vi "运维调试_CODCr.vi"() -> ()   [LabVIEW 2016, in "CodCr.lvlib"]
uses:
  CodCr.lvlib
  <vilib>/Utility/miscctls.llb/LVPointTypeDef.ctl
  <vilib>/Plasmionique/MB Master/MB_Master_Serial/MB_Master_Serial.lvclass
  C:/Program Files (x86)/National Instruments/LabVIEW 2016/vi.lib/Plasmionique/MB Master/MB_Master/MB_Master.lvclass
  <vilib>/Plasmionique/MB Master/MB Master.lvlib
  <vilib>/ptbypt/NI_PtbyPt.lvlib
panel:
  out "COM口":string
  in  "空白测试":bool
  in  "隐藏按钮":bool
  in  "写入消解温度时长":bool
  in  "保存KB值":bool
  out "source":string
  in  "标样核查":bool
  out "启动时间":timestamp format="%<%Y/%m/%d %H:%M:%S>T"
  out "主循环次数":i32
  out "status":bool
  out "启动测量模式":T1(ring)
  out "曲线斜率B":sgl format="%#_10g"
  out "曲线斜率K":sgl format="%#_10g"
  out "量程上限":sgl
  out "量程下限":sgl
  out "消解时长":u16
  out "消解温度":u16
  out "测量精度":u16
  out "测量结果":sgl
  out "标样参考值":sgl
  out "量程":u16
  out "工作状态":T1(ring)
  out "仪器时间":timestamp format="%<%X\n%x>T"
  out "关键参数区":T2
  out "状态告警区":T3
  out "测量数据区":T4 {"单位" items=["ug/L", "mg/L", "ppm", "mg/m3", "cm", "ppb", "ug/m3", "%", "nmol/mol", "umol/mol", "MPN/L", "MPN/100ml", "ng/m3", "NTU", "无量纲", "ms/cm", "us/cm", "℃", "mV", "万个/L"]}
  out "系统时间":timestamp format="%<%Y/%m/%d %H:%M:%S>T"
  in  "VISA Resource":refnum<visa-resource-name>="COM9"
  out "Registers":u16[](array[numeric])
  in  "枚举":enum16{"读取", "写入", "读取参数"}(ring)
  in  "停止":bool
  in  "校时":bool
  in  "标样校准":bool
  in  "空白校准":bool
  in  "零点核查":bool
  in  "跨度核查":bool
  in  "水样测试":bool
  in  "返回":bool
  in  "设置":bool
  # "mg/L"
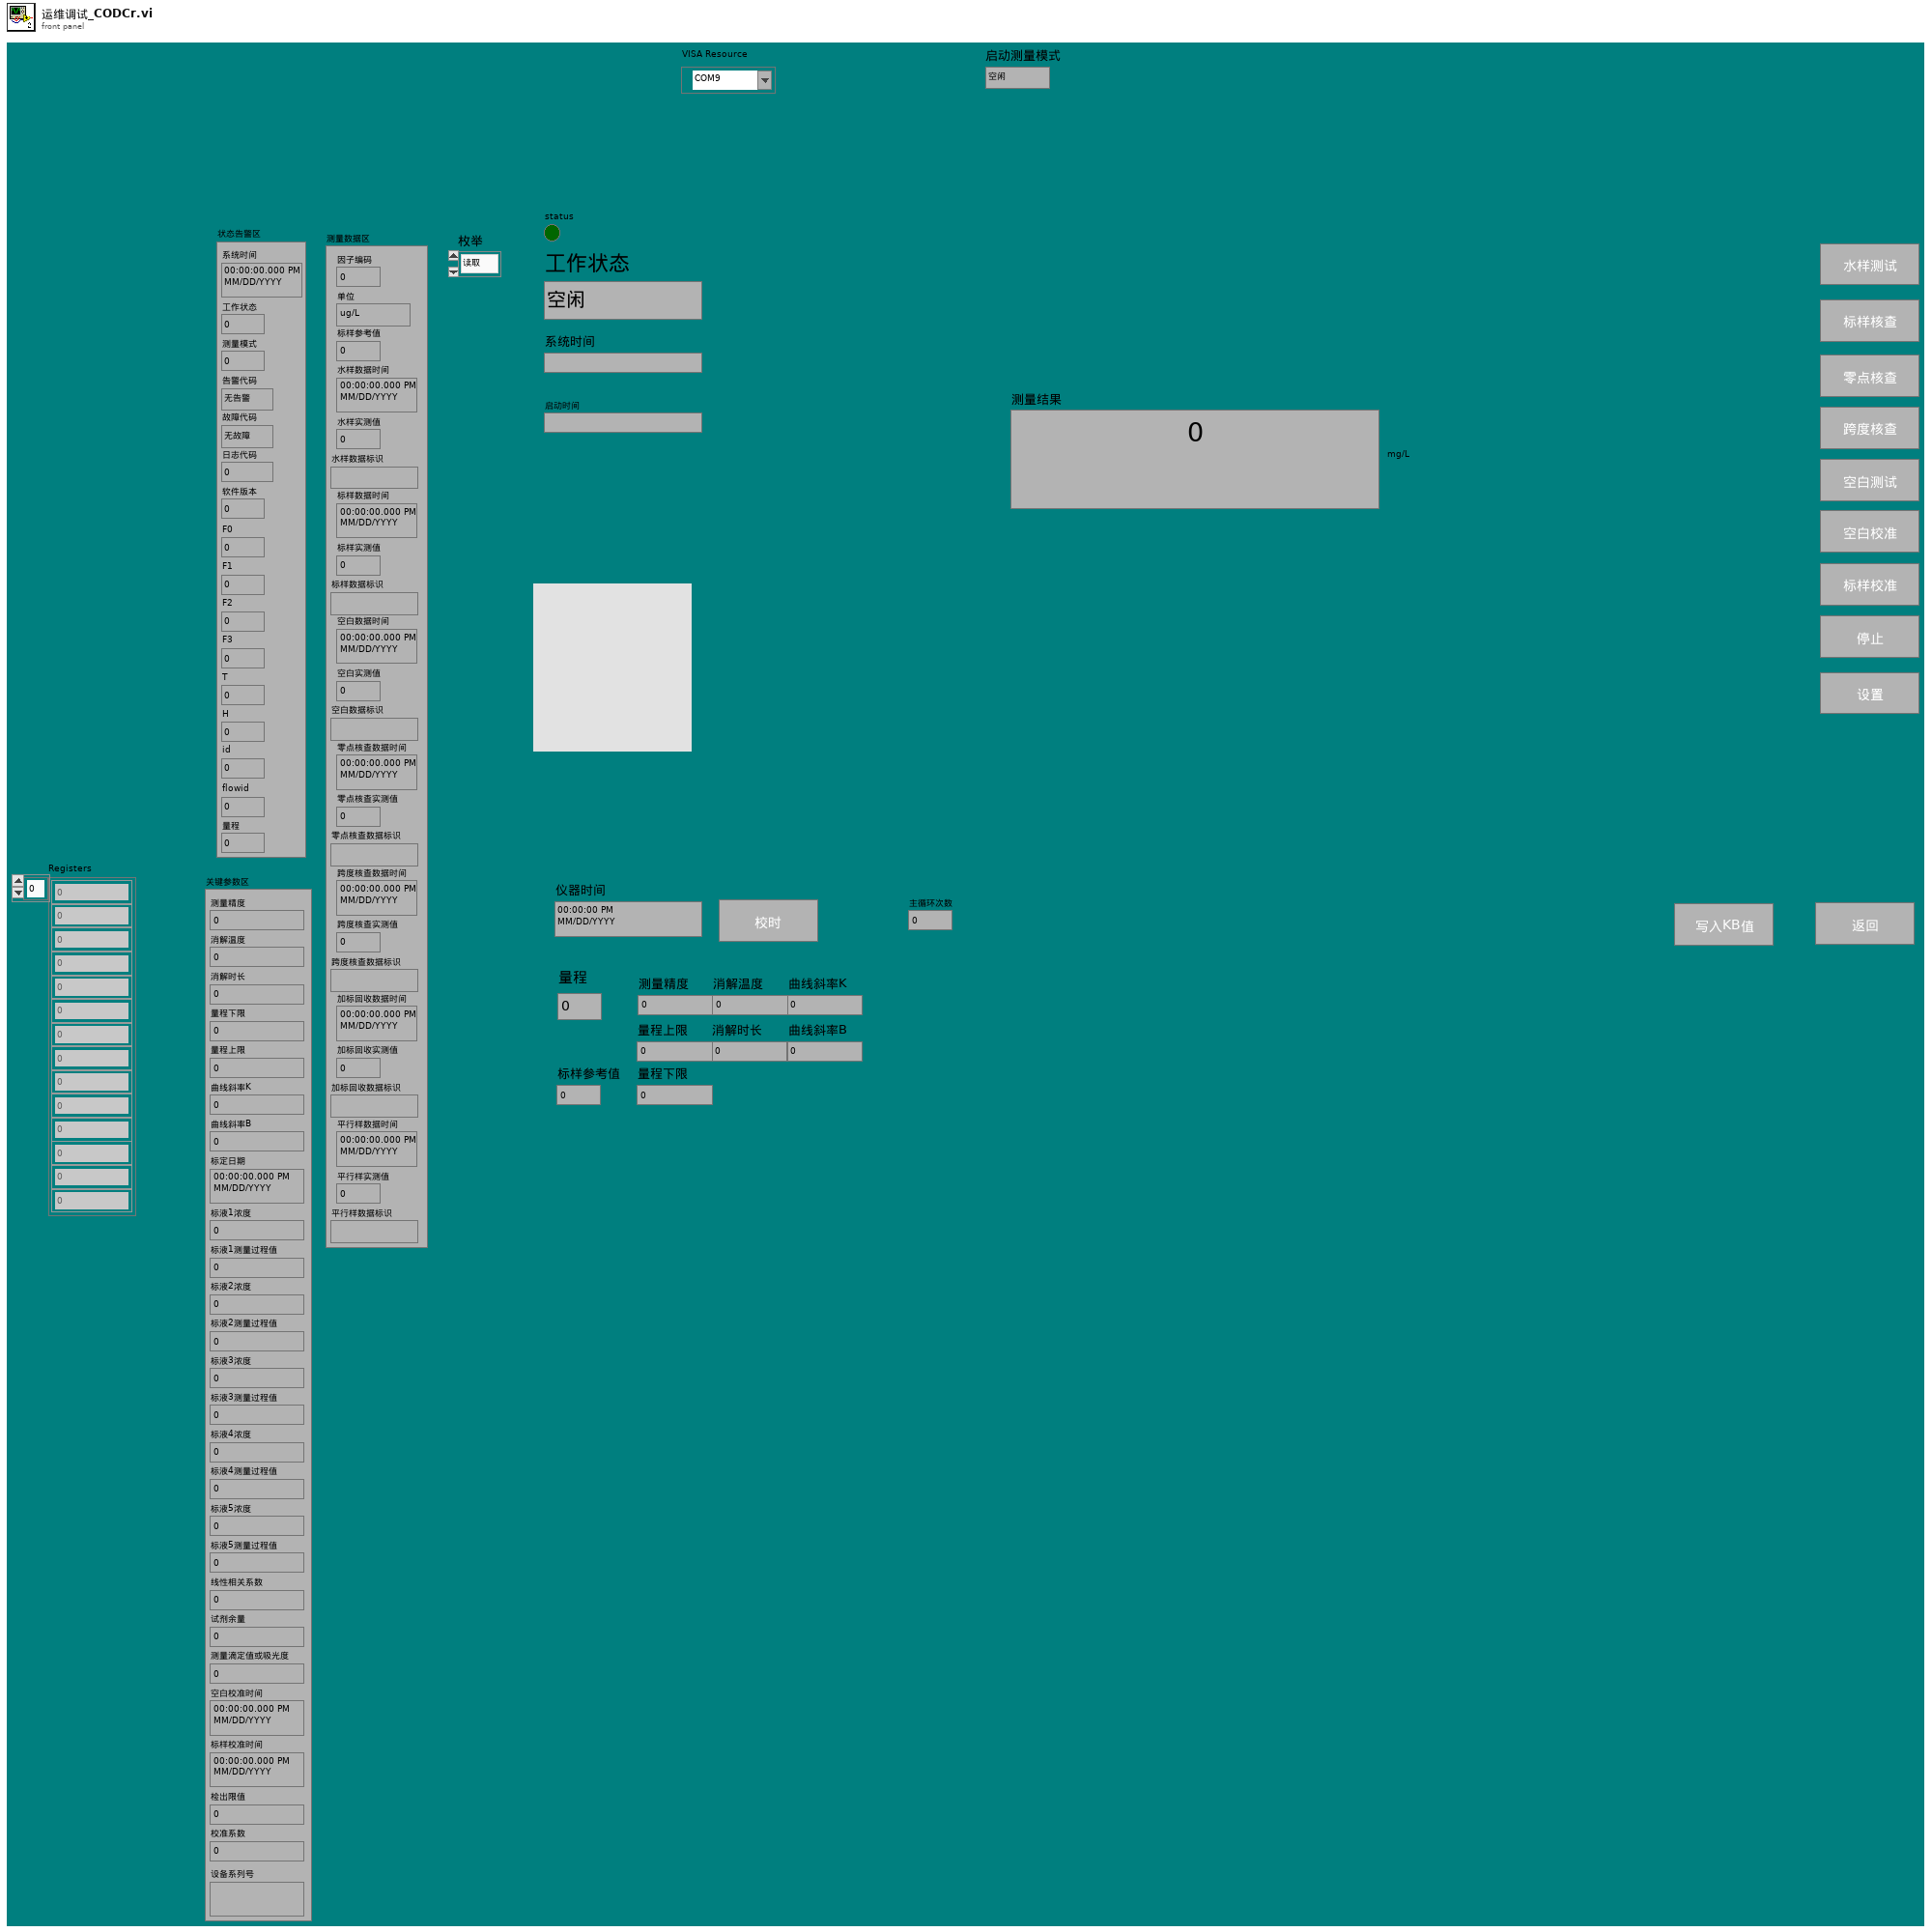
[diagram p1: front panel]
types:
  T1 = enum16{"空闲", "水样测试", "标样核查", "零点核查", "跨度核查", "空白测试", "平行样测试", "加标回收", "空白校准", "标样校准", "初始化（清洗）"}
  T2 = cluster{"测量精度":u16, "消解温度":u16, "消解时长":u16, "量程下限":sgl, "量程上限":sgl, "曲线斜率K":sgl, "曲线斜率B":sgl, "标定日期":timestamp, "标液1浓度":sgl, "标液1测量过程值":sgl, "标液2浓度":sgl, "标液2测量过程值":sgl, "标液3浓度":sgl, "标液3测量过程值":sgl, "标液4浓度":sgl, "标液4测量过程值":sgl, "标液5浓度":sgl, "标液5测量过程值":sgl, "线性相关系数":sgl, "试剂余量":u32, "测量滴定值或吸光度":sgl, "空白校准时间":timestamp, "标样校准时间":timestamp, "检出限值":sgl, "校准系数":sgl, "设备系列号":string}
  T3 = cluster{"系统时间":timestamp, "工作状态":u16, "测量模式":u16, "告警代码":enum16{"无告警", "缺试剂告警", "缺水样告警", "缺蒸馏水告警", "缺标液告警", "仪表漏液告警", "标定异常告警", "超量程告警", "加热异常", "低试剂预警", "超上限告警", "超下限告警", "仪表内部其他异常", "滴定异常告警", "电极异常告警", "量程切换告警", "参数设置告警", "PH电极电位异常", "电导率电极异常", "浊度光度异常", "溶解氧电极异常", "溶解氧光强异常", "温度异常告警", "PH异常告警", "溶解氧异常告警", "电导率异常告警", "浊度异常告警", "叶绿素异常告警", "藻密度异常告警", "蓝绿藻异常告警", "ORP异常告警", "氨氮异常告警", "清洁刷异常告警", "SD卡异常告警", "蓝牙异常告警", "Wifi异常告警", "流程异常告警"}, "故障代码":enum16{"无故障", "电机故障", "温度故障", "通讯故障", "滴定故障"}, "日志代码":u16, "软件版本":u16, "F0":sgl, "F1":sgl, "F2":sgl, "F3":sgl, "T":sgl, "H":sgl, "id":u16, "flowid":u16, "量程":u16}
  T4 = cluster{"因子编码":u32, "单位":u16, "标样参考值":sgl, "水样数据时间":timestamp, "水样实测值":sgl, "水样数据标识":string, "标样数据时间":timestamp, "标样实测值":sgl, "标样数据标识":string, "空白数据时间":timestamp, "空白实测值":sgl, "空白数据标识":string, "零点核查数据时间":timestamp, "零点核查实测值":sgl, "零点核查数据标识":string, "跨度核查数据时间":timestamp, "跨度核查实测值":sgl, "跨度核查数据标识":string, "加标回收数据时间":timestamp, "加标回收实测值":sgl, "加标回收数据标识":string, "平行样数据时间":timestamp, "平行样实测值":sgl, "平行样数据标识":string}
  T5 = cluster{"baud rate (bps)":u32, "stop bits":u16, "parity":u16, "flow control":u16, "timeout":u32, "retries":i32}
  T6 = cluster{"starting address":u16, "number of holding registers":u16}
  T7 = typedef "LVPointTypeDef.ctl" = cluster{"Horizontal":i16, "Vertical":i16}
  T8 = cluster{"时间标识":timestamp, "监测值":sgl, "单位":u16, "数据标识":string, "因子编码":u32, "标样参考值":sgl, "F0":sgl, "F1":sgl, "F2":sgl, "F3":sgl, "温度":sgl, "湿度":sgl, "量程标识":string}
  T9 = cluster{"系统时间":timestamp, "工作状态":enum16{"空闲", "水样测试", "标样核查", "零点核查", "跨度核查", "空白测试", "平行样测试", "加标回收", "空白校准", "标样校准", "初始化（清洗）"}, "测量模式":enum16{"待机", "连续模式", "周期模式", "定点模式", "受控模式", "手动模式"}, "告警代码":enum16{"无告警", "缺试剂告警", "缺水样告警", "缺蒸馏水告警", "缺标液告警", "仪表漏液告警", "标定异常告警", "超量程告警", "加热异常", "低试剂预警", "超上限告警", "超下限告警", "仪表内部其他异常", "滴定异常告警", "电极异常告警", "量程切换告警", "参数设置告警", "PH电极电位异常", "电导率电极异常", "浊度光度异常", "溶解氧电极异常", "溶解氧光强异常", "温度异常告警", "PH异常告警", "溶解氧异常告警", "电导率异常告警", "浊度异常告警", "叶绿素异常告警", "藻密度异常告警", "蓝绿藻异常告警", "ORP异常告警", "氨氮异常告警", "清洁刷异常告警", "SD卡异常告警", "蓝牙异常告警", "Wifi异常告警", "流程异常告警"}, "故障代码":enum16{"无故障", "电机故障", "温度故障", "通讯故障", "滴定故障"}, "日志代码":u16, "软件版本":u16, "F0":sgl, "F1":sgl, "F2":sgl, "F3":sgl, "T":sgl, "H":sgl, "id":u16, "flowid":u16, "量程":u16}
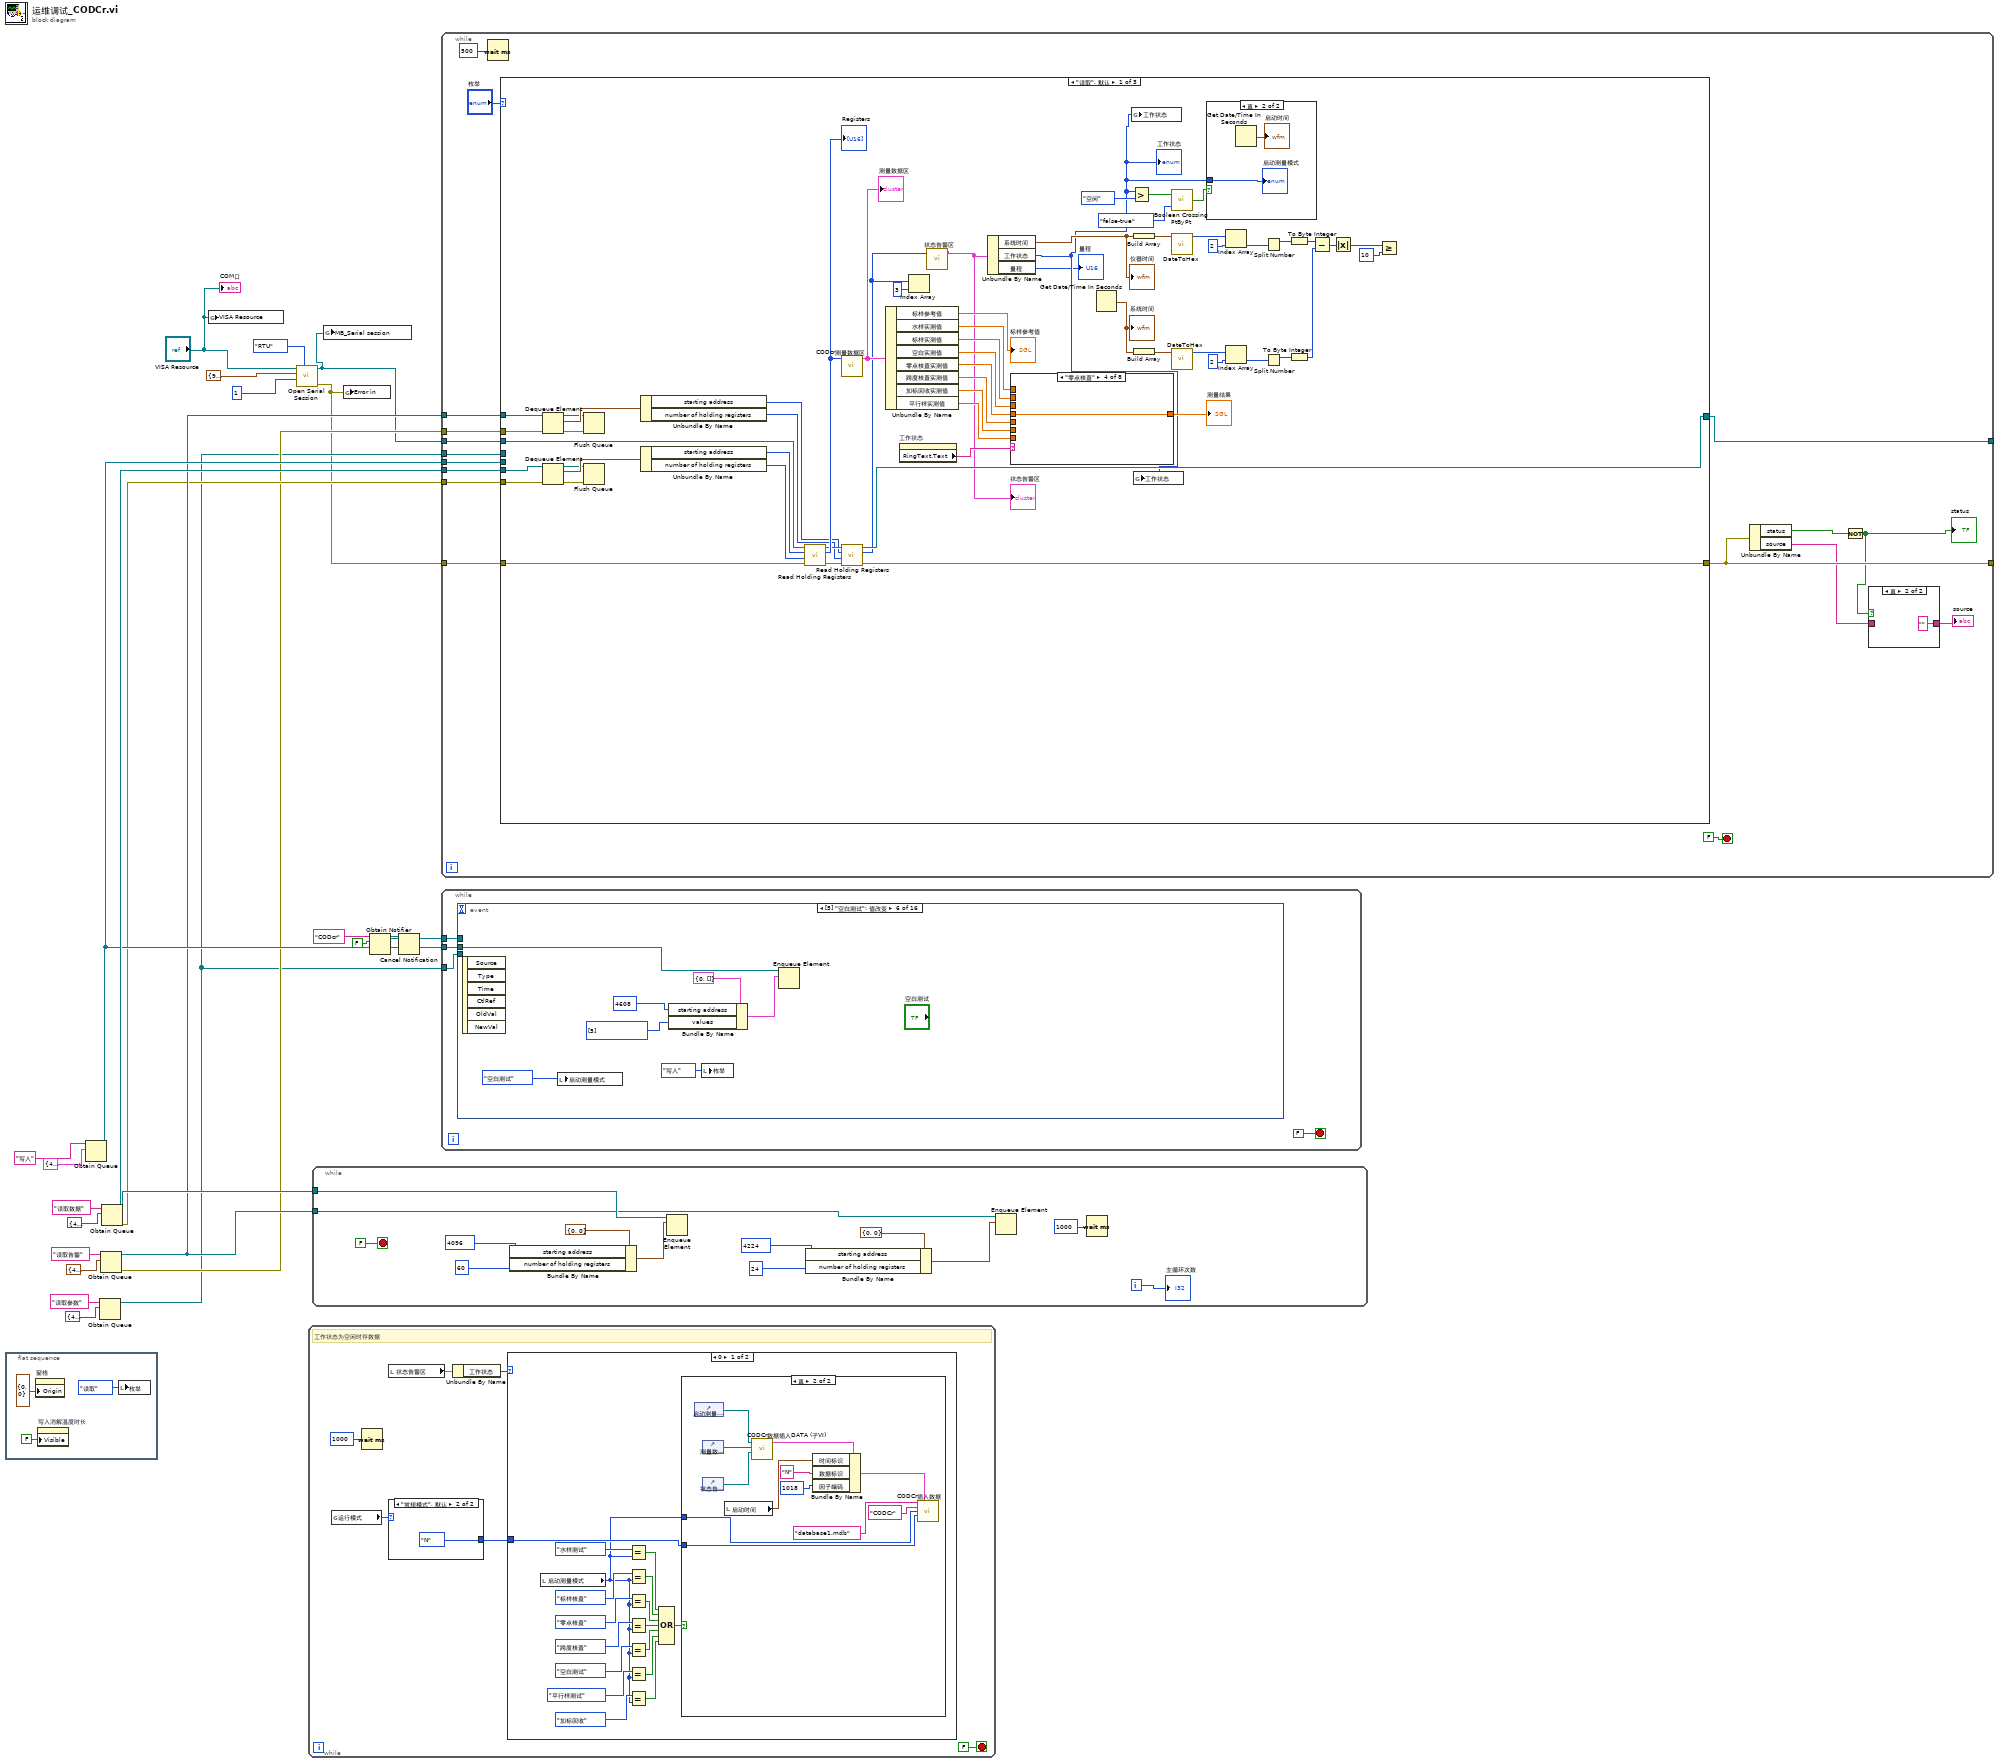
[diagram p0: block diagram]
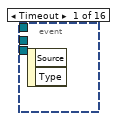
[diagram p2: hidden frame]
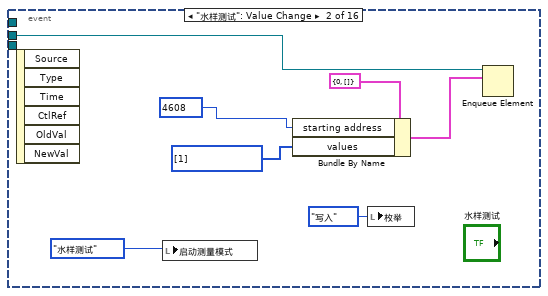
[diagram p3: hidden frame]
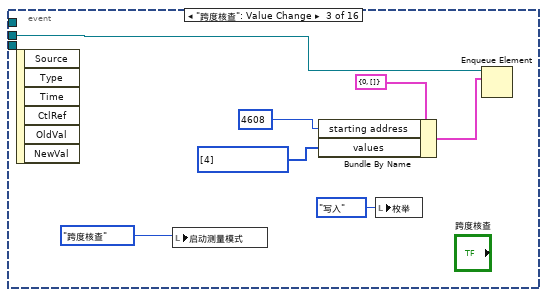
[diagram p4: hidden frame]
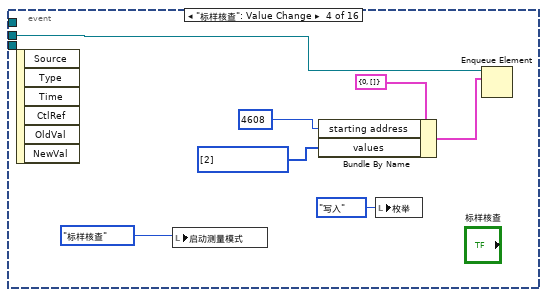
[diagram p5: hidden frame]
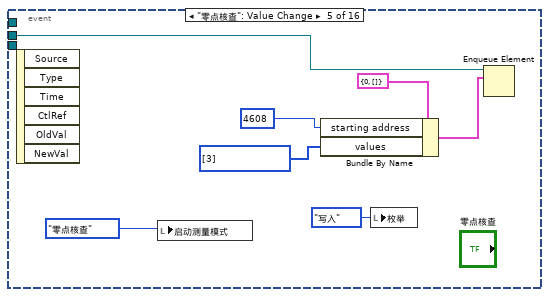
[diagram p6: hidden frame]
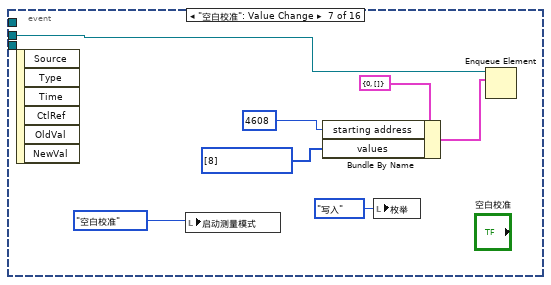
[diagram p7: hidden frame]
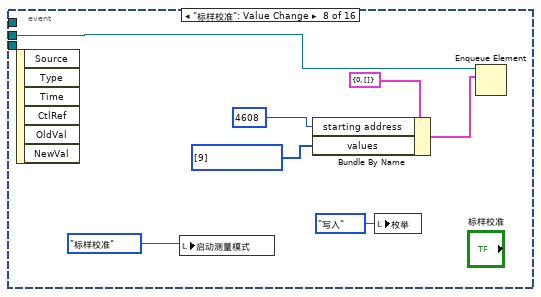
[diagram p8: hidden frame]
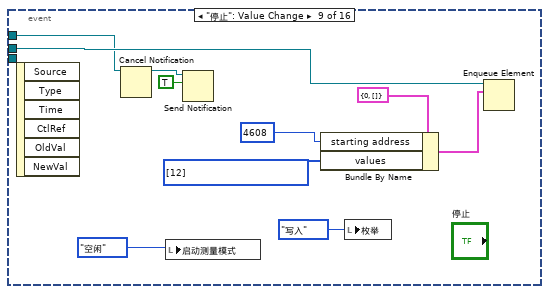
[diagram p9: hidden frame]
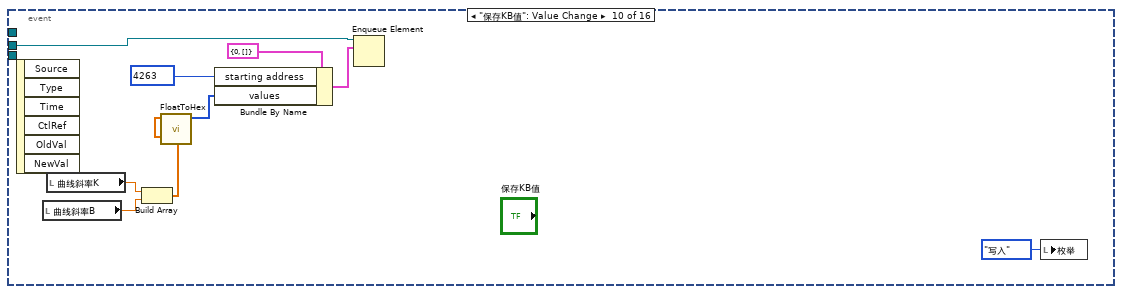
[diagram p10: hidden frame]
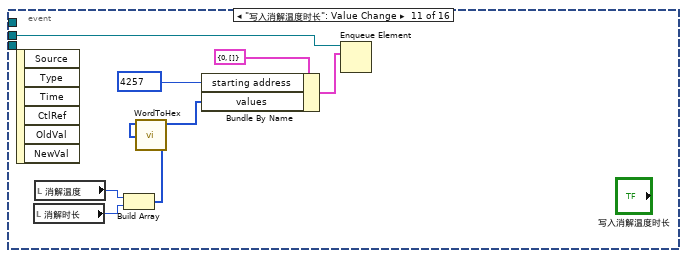
[diagram p11: hidden frame]
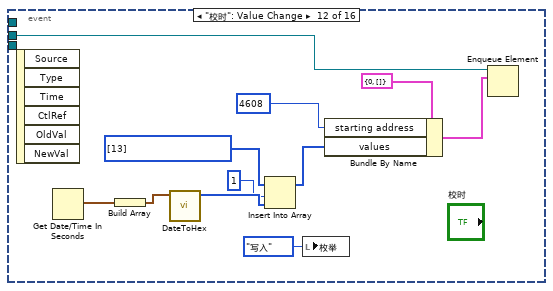
[diagram p12: hidden frame]
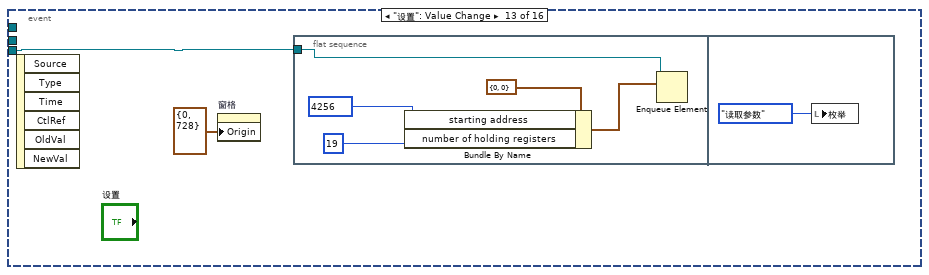
[diagram p13: hidden frame]
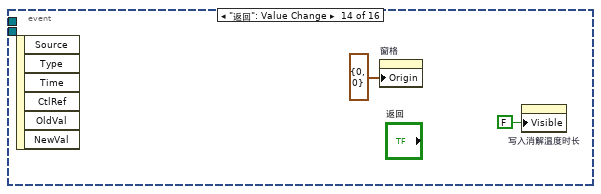
[diagram p14: hidden frame]
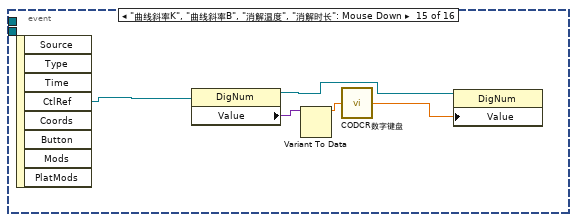
[diagram p15: hidden frame]
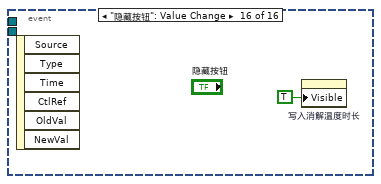
[diagram p16: hidden frame]
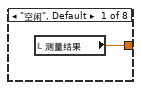
[diagram p18: hidden frame]
diagram:
  n1 = flat-sequence {
    frame #0 {
      n2 = property on="窗格" class="Pane"("Origin"=T7 {"Horizontal"=0, "Vertical"=0} ("原点")) -> ()  [unwired: 2 in, 2 out]
      n3 = property on="写入消解温度时长" class="Bool"("Visible"=FALSE ("可见")) -> ()  [unwired: 2 in, 2 out]
      n4 = local write "枚举"(enum16{"读取", "写入", "读取参数"}."读取" ("枚举")) -> ()
    }
  }
  n5 = Obtain Queue(name (unnamed)="写入" ("名称（未命名）"), element data type=cluster{"starting address":u16, "values":u16[]} {"starting address"=4096, "values"=[]}) -> (queue out=w16:refnum<queue>)  [unwired: 3 in, 2 out]
  n6 = Obtain Queue(name (unnamed)="读取参数" ("名称（未命名）"), element data type=T6 {"starting address"=4096, "number of holding registers"=100}) -> (queue out=w4:refnum<queue>)  [unwired: 3 in, 2 out]
  n7 = Obtain Queue(name (unnamed)="读取告警" ("名称（未命名）"), element data type=T6 {"starting address"=4096, "number of holding registers"=100}) -> (queue out=w13:refnum<queue>, error out=w9:errorcluster)  [unwired: 3 in, 1 out]
  n8 = Obtain Queue(name (unnamed)="读取数据" ("名称（未命名）"), element data type=T6 {"starting address"=4096, "number of holding registers"=100}) -> (queue out=w17:refnum<queue>, error out=w10:errorcluster)  [unwired: 3 in, 1 out]
  n9 = global write "CODcr全局变量.vi" "VISA Resource"("VISA Resource") -> ()
  n10 = call <vilib>:"Open Serial Session.vi"("Mode (RTU)"=enum16{"RTU", "ASCII"}."RTU", "Slave ID"=u8 1, "Serial Config"=T5 {"baud rate (bps)"=9600, "stop bits"=10, "parity"=0, "flow control"=0, "timeout"=1000, "retries"=1}, "VISA Resource"="VISA Resource") -> ("Error out"=w1:errorcluster, "MB_Serial session"=w2:refnum<class "MB_Master_Serial.lvclass">)  [unwired: 6 in]
  n11 = while "While循环" {
    stop <- FALSE stop-if-true
    # "工作状态为空闲时存数据"
    n12 = global read "系统变量.vi" "运行模式"() -> (w29:enum16{"维护模式", "常规模式", "应急模式", "质控模式"})
    n13 = Wait (ms)(milliseconds to wait=u32 1000 ("等待时间（毫秒）")) -> ()  [unwired: 1 out]
    n14 = local read "状态告警区"() -> (w31:T3)
    n15 = case shown="\"常规模式\", 默认" w29 {
      tunnel: [enum16{"N", "M"}."M" ("数据类型") enum16{"N", "M"}."N" ("数据类型")] -> w28
      frame "维护模式" {
      }
      frame "常规模式", Default {
      }
    }
    n16 = Unbundle By Name(w31) -> ("工作状态"=w30:u16)
    n17 = case shown="0" w30 {
      tunnel: w28 -> [w52 _]
      frame 0 {
        n18 = local read "启动测量模式"() -> (w44:T1)
        n19 = Equal?(x=T1."水样测试" ("启动测量模式"), y=w44) -> (x = y?=w43:bool)
        n20 = Equal?(x=T1."标样核查" ("启动测量模式"), y=w44) -> (x = y?=w42:bool)
        n21 = Equal?(x=T1."零点核查" ("启动测量模式"), y=w44) -> (x = y?=w41:bool)
        n22 = Equal?(x=T1."跨度核查" ("启动测量模式"), y=w44) -> (x = y?=w40:bool)
        n23 = Equal?(x=T1."空白测试" ("启动测量模式"), y=w44) -> (x = y?=w39:bool)
        n24 = Equal?(x=T1."平行样测试" ("启动测量模式"), y=w44) -> (x = y?=w38:bool)
        n25 = Equal?(x=T1."加标回收" ("启动测量模式"), y=w44) -> (x = y?=w37:bool)
        n26 = Compound Arithmetic op=OR(w43, w42, w41, w40, w39, w38, w37) -> (w36:bool)
        n27 = case shown="真" w36 {
          tunnel: w44 -> [_ w62]
          tunnel: w52 -> [_ w61]
          frame False {
          }
          frame True {
            n28 = control-ref of="启动测量模式"() -> (w60:refnum<vi>)
            n29 = control-ref of="测量数据区"() -> (w59:refnum<vi>)
            n30 = control-ref of="状态告警区"() -> (w58:refnum<vi>)
            n31 = local read "启动时间"() -> (w56:timestamp)
            n32 = call "CODCr数据插入DATA (子VI).vi"("reference 2"=w58, "reference"=w59, "Enum输入"=w60) -> ("data"=w57:T8)  [unwired: 8 in]
            n33 = Bundle By Name(cluster=w57, "时间标识"=w56, "数据标识"="N", "因子编码"=u32 1018) -> (w55:T8)
            n34 = call "CODCr插入数据.vi"("database"="database1.mdb", "data"=w55, "table"="CODCr", "测量模式"=w62, "数据类型"=w61) -> ()  [unwired: 10 in, 1 out]
          }
        }
      }
      frame 1, Default {
      }
    }
  }
  n35 = while {
    tunnel: w17 -> [w75]
    tunnel: w13 -> [w66]
    i -> [w65]
    stop <- FALSE stop-if-true
    n36 = Bundle By Name(cluster=T6 {"starting address"=0, "number of holding registers"=0} ("元素"), "starting address"=u16 4096, "number of holding registers"=u16 60) -> (w73:T6)
    n37 = Enqueue Element(queue=w75, element=w73) -> ()  [unwired: 2 in, 3 out]
    n38 = Bundle By Name(cluster=T6 {"starting address"=0, "number of holding registers"=0} ("元素"), "starting address"=u16 4224, "number of holding registers"=u16 24) -> (w67:T6)
    n39 = Enqueue Element(queue=w66, element=w67) -> ()  [unwired: 2 in, 3 out]
    n40 = Wait (ms)(milliseconds to wait=u32 1000 ("等待时间（毫秒）")) -> ()  [unwired: 1 out]
    "主循环次数" <- w65
  }
  n41 = global write "CODcr全局变量.vi" "MB_Serial session"(w2) -> ()
  n42 = global write "CODcr全局变量.vi" "Error in"(w1) -> ()
  n43 = Obtain Notifier(name (unnamed)="CODcr" ("名称（未命名）"), notification data type=FALSE) -> (notifier out=w5:refnum<notifier>)  [unwired: 2 in, 2 out]
  n44 = Cancel Notification(0:w5) -> (8:w6:refnum<notifier>)  [unwired: 1 in, 2 out]
  n45 = while {
    tunnel: w16 -> [w91]
    tunnel: w17 -> [w90]
    tunnel: w13 -> [w89]
    tunnel: w4 -> [w88]
    tunnel: w10 -> [w86]
    tunnel: w9 -> [w85]
    tunnel: w1 -> [w84]
    tunnel: [w82] -> _
    tunnel: w2 -> [w92]
    tunnel: [w87] -> _
    stop <- FALSE stop-if-true
    n46 = Wait (ms)(milliseconds to wait=u32 500 ("等待时间（毫秒）")) -> ()  [unwired: 1 out]
    n47 = case shown="\"读取\", 默认" "枚举" {
      tunnel: w92 -> [w154 w171 w194]
      tunnel: w84 -> [w130 w170 w193]
      tunnel: w91 -> [_ w169 _]
      tunnel: w90 -> [w153 _ _]
      tunnel: w89 -> [w148 _ _]
      tunnel: w88 -> [_ _ w195]
      tunnel: [w129 w165 w183] -> w82
      tunnel: [w111 w166 w184] -> w87
      tunnel: w86 -> [w105 _ _]
      tunnel: w85 -> [w102 _ _]
      frame "读取", Default {
        n48 = Dequeue Element(queue=w148, error in (no error)=w102) -> (queue out=w104:refnum<queue>, element=w147:T6, error out=w103:errorcluster)  [unwired: 1 in, 1 out]
        n49 = Dequeue Element(queue=w153, error in (no error)=w105) -> (queue out=w107:refnum<queue>, element=w152:T6, error out=w106:errorcluster)  [unwired: 1 in, 1 out]
        n50 = Flush Queue(queue=w104, error in (no error)=w103) -> ()  [unwired: 3 out]
        n51 = Flush Queue(queue=w107, error in (no error)=w106) -> ()  [unwired: 3 out]
        n52 = Unbundle By Name(w147) -> ("starting address"=w144:u16, "number of holding registers"=w143:u16)
        n53 = Unbundle By Name(w152) -> ("starting address"=w151:u16, "number of holding registers"=w150:u16)
        n54 = call <vilib>:"Read Holding Registers.vi"("error in (no error)"=w130, "quantity"=w150, "starting address"=w151, "MB session in"=w154) -> ("error out"=w145:errorcluster, "Registers"=w149:u16[], "MB session out"=w146:refnum<class "MB_Master_Serial.lvclass">)  [unwired: 5 in]
        "Registers" <- w149
        n55 = call "CODcr测量数据区.vi"("数组"=w149) -> ("测量数据区"=w142:T4)  [unwired: 10 in]
        "测量数据区" <- w142
        n56 = call <vilib>:"Read Holding Registers.vi"("error in (no error)"=w145, "quantity"=w143, "starting address"=w144, "MB session in"=w146) -> ("error out"=w129:errorcluster, "Registers"=w98:u16[], "MB session out"=w111:refnum<class "MB_Master_Serial.lvclass">)  [unwired: 5 in]
        n57 = Unbundle By Name(w142) -> ("标样参考值"=→"标样参考值":sgl, "水样实测值"=w138:sgl, "标样实测值"=w136:sgl, "空白实测值"=w133:sgl, "零点核查实测值"=w135:sgl, "跨度核查实测值"=w134:sgl, "加标回收实测值"=w131:sgl, "平行样实测值"=w132:sgl)
        n58 = property on="工作状态" class="Enum (严格)"() -> ("RingText.Text"=w139:string)  [unwired: 2 in, 2 out]
        n59 = Index Array(array=w98, index=3 ("索引")) -> ()  [unwired: 1 out]
        n60 = call "状态告警区.vi"("数组"=w98) -> ("状态告警区"=w97:T9)  [unwired: 10 in]
        "状态告警区" <- w97
        n61 = Unbundle By Name(w97) -> ("系统时间"=w112:timestamp, "工作状态"=w100:T1, "量程"=→"量程":u16)
        "仪器时间" <- w112
        "工作状态" <- w100
        n62 = case shown="\"零点核查\"" w139 {
          tunnel: w138 -> [_ w156 _ _ _ _ _ _]
          tunnel: [w155 w156 w157 w158 w159 w160 w161 w162] -> w137
          tunnel: w136 -> [_ _ w157 _ _ _ _ _]
          tunnel: w135 -> [_ _ _ w158 _ _ _ _]
          tunnel: w134 -> [_ _ _ _ w159 _ _ _]
          tunnel: w133 -> [_ _ _ _ _ w160 _ _]
          tunnel: w132 -> [_ _ _ _ _ _ w161 _]
          tunnel: w131 -> [_ _ _ _ _ _ _ w162]
          frame "空闲", Default {
            n63 = local read "测量结果"() -> (w155:sgl)
          }
          frame "水样测试" {
          }
          frame "标样核查" {
          }
          frame "零点核查" {
          }
          frame "跨度核查" {
          }
          frame "空白测试" {
          }
          frame "平行样测试" {
          }
          frame "加标回收" {
          }
        }
        "测量结果" <- w137
        n64 = Get Date/Time In Seconds() -> (seconds since 1Jan1904=w114:timestamp)
        "系统时间" <- w114
        n65 = Greater?(x=w100, y=T1."空闲") -> (0:w110:bool)
        n66 = global write "CODcr全局变量.vi" "工作状态"(w100) -> ()
        n67 = Build Array(w112) -> (w128:timestamp[])
        n68 = Build Array(w114) -> (w113:timestamp[])
        n69 = global write "CODCr工作状态.vi" "工作状态"(w100) -> ()
        n70 = call <vilib>:"Boolean Crossing PtByPt.vi"("direction"=enum16{"either", "false-true", "true-false"}."false-true", "input"=w110) -> ("crossing"=w109:bool)  [unwired: 1 in]
        n71 = call "DateToHex.vi"("DATE"=w128) -> ("数组"=w120:u16[])  [unwired: 10 in]
        n72 = call "DateToHex.vi"("DATE"=w113) -> ("数组"=w115:u16[])  [unwired: 10 in]
        n73 = case shown="真" w109 {
          tunnel: w100 -> [_ w163]
          frame False {
          }
          frame True {
            n74 = Get Date/Time In Seconds() -> (seconds since 1Jan1904=→"启动时间":timestamp)
            "启动测量模式" <- w163
          }
        }
        n75 = Index Array(array=w120, index=2 ("索引")) -> (element=w118:u16)
        n76 = Index Array(array=w115, index=2 ("索引")) -> (element=w117:u16)
        n77 = Split Number(x=w118) -> (hi(x)=w124:u8)  [unwired: 1 out]
        n78 = Split Number(x=w117) -> (hi(x)=w121:u8)  [unwired: 1 out]
        n79 = To Byte Integer(number=w124) -> (8bit integer=w125:i8)
        n80 = To Byte Integer(number=w121) -> (8bit integer=w122:i8)
        n81 = Subtract(x=w125, y=w122) -> (x-y=w123:i8)
        n82 = Absolute Value(x=w123) -> (abs(x)=w126:i8)
        n83 = Greater Or Equal?(x=w126, y=i8 10) -> ()  [unwired: 1 out]
      }
      frame "写入" {
        n84 = flat-sequence {
          tunnel: w171 -> [w179]
          tunnel: w170 -> [w178]
          tunnel: w169 -> [w175]
          tunnel: [w177] -> w168
          tunnel: [w176] -> w167
          tunnel: w168 -> [w181]
          tunnel: w167 -> [w180]
          tunnel: [w181] -> w166
          tunnel: [w180] -> w165
          frame #0 {
            n85 = Dequeue Element(queue=w175) -> (element=w174:cluster{"starting address":u16, "values":u16[]})  [unwired: 2 in, 3 out]
            n86 = Unbundle By Name(w174) -> ("starting address"=w173:u16, "values"=w172:u16[])
            n87 = call <vilib>:"Write Multiple Registers.vi"("error in (no error)"=w178, "values"=w172, "starting address"=w173, "MB session in"=w179) -> ("error out"=w176:errorcluster, "MB session out"=w177:refnum<class "MB_Master_Serial.lvclass">)  [unwired: 6 in]
          }
          frame #1 {
            n88 = local write "枚举"(enum16{"读取", "写入", "读取参数"}."读取" ("枚举")) -> ()
          }
        }
      }
      frame "读取参数" {
        n89 = local write "枚举"(enum16{"读取", "写入", "读取参数"}."读取" ("枚举")) -> ()
        n90 = Dequeue Element(queue=w195, timeout in ms (-1)=1000 ("超时毫秒(-1)")) -> (element=w202:T6)  [unwired: 1 in, 3 out]
        n91 = Unbundle By Name(w202) -> ("starting address"=w201:u16, "number of holding registers"=w200:u16)
        n92 = call <vilib>:"Read Holding Registers.vi"("error in (no error)"=w193, "quantity"=w200, "starting address"=w201, "MB session in"=w194) -> ("error out"=w197:errorcluster, "Registers"=w199:u16[], "MB session out"=w184:refnum<class "MB_Master_Serial.lvclass">)  [unwired: 5 in]
        n93 = call "关键参数区.vi"("数组"=w199) -> ("关键参数区"=w196:T2)  [unwired: 10 in]
        "关键参数区" <- w196
        n94 = Unbundle By Name(w196) -> ("测量精度"=→"测量精度":u16, "消解温度"=→"消解温度":u16, "消解时长"=→"消解时长":u16, "量程下限"=→"量程下限":sgl, "量程上限"=→"量程上限":sgl, "曲线斜率K"=→"曲线斜率K":sgl, "曲线斜率B"=→"曲线斜率B":sgl)
        n95 = call <vilib>:"Clear Errors.vi"("error in (no error)"=w197) -> ("error out"=w183:errorcluster)  [unwired: 5 in, 1 out]
      }
    }
    n96 = Unbundle By Name(w82) -> ("status"=w83:bool, "source"=w80:string)
    n97 = Not(x=w83) -> (.not. x?=w79:bool)
    "status" <- w79
    n98 = case shown="真" w79 {
      tunnel: w80 -> [w95 _]
      tunnel: [w95 "" ("source")] -> w78
      frame False {
      }
      frame True {
      }
    }
    "source" <- w78
  }
  n99 = while {
    tunnel: w16 -> [w205]
    tunnel: w6 -> [w204]
    tunnel: w4 -> [w203]
    stop <- FALSE stop-if-true
    n100 = event shown="[5] \"空白测试\": 值改变" {
      selector: _ -> [_ _ _ _ _ _ _ _ _ _ _ _ _ _ _ _]
      dyn-events: _ -> [_ _ _ _ _ _ _ _ _ _ _ _ _ _ _ _]
      timeout: _ -> [_ _ _ _ _ _ _ _ _ _ _ _ _ _ _ _]
      tunnel: w205 -> [_ w213 w216 w223 w230 w237 w244 w251 w261 w273 w279 w290 _ _ _ _]
      tunnel: w204 -> [_ _ _ _ _ _ _ _ w259 _ _ _ _ _ _ _]
      tunnel: w203 -> [_ _ _ _ _ _ _ _ _ _ _ _ w294 _ _ _]
      event Timeout {
        n101 = event-data() -> ()  [unwired: 1 in, 2 out]
      }
      event "水样测试": Value Change {
        n102 = event-data() -> ()  [unwired: 1 in, 6 out]
        n103 = local write "启动测量模式"(T1."水样测试" ("启动测量模式")) -> ()
        n104 = Bundle By Name(cluster=cluster{"starting address":u16, "values":u16[]} {"starting address"=0, "values"=[]} ("元素"), "starting address"=u16 4608, "values"=u16[] [1]) -> (w211:cluster{"starting address":u16, "values":u16[]})
        n105 = local write "枚举"(enum16{"读取", "写入", "读取参数"}."写入" ("枚举")) -> ()
        n106 = Enqueue Element(queue=w213, element=w211) -> ()  [unwired: 2 in, 3 out]
      }
      event "跨度核查": Value Change {
        n107 = event-data() -> ()  [unwired: 1 in, 6 out]
        n108 = local write "启动测量模式"(T1."跨度核查" ("启动测量模式")) -> ()
        n109 = Bundle By Name(cluster=cluster{"starting address":u16, "values":u16[]} {"starting address"=0, "values"=[]} ("元素"), "starting address"=u16 4608, "values"=u16[] [4]) -> (w219:cluster{"starting address":u16, "values":u16[]})
        n110 = local write "枚举"(enum16{"读取", "写入", "读取参数"}."写入" ("枚举")) -> ()
        n111 = Enqueue Element(queue=w216, element=w219) -> ()  [unwired: 2 in, 3 out]
      }
      event "标样核查": Value Change {
        n112 = event-data() -> ()  [unwired: 1 in, 6 out]
        n113 = local write "启动测量模式"(T1."标样核查" ("启动测量模式")) -> ()
        n114 = Bundle By Name(cluster=cluster{"starting address":u16, "values":u16[]} {"starting address"=0, "values"=[]} ("元素"), "starting address"=u16 4608, "values"=u16[] [2]) -> (w226:cluster{"starting address":u16, "values":u16[]})
        n115 = local write "枚举"(enum16{"读取", "写入", "读取参数"}."写入" ("枚举")) -> ()
        n116 = Enqueue Element(queue=w223, element=w226) -> ()  [unwired: 2 in, 3 out]
      }
      event "零点核查": Value Change {
        n117 = event-data() -> ()  [unwired: 1 in, 6 out]
        n118 = local write "启动测量模式"(T1."零点核查" ("启动测量模式")) -> ()
        n119 = Bundle By Name(cluster=cluster{"starting address":u16, "values":u16[]} {"starting address"=0, "values"=[]} ("元素"), "starting address"=u16 4608, "values"=u16[] [3]) -> (w233:cluster{"starting address":u16, "values":u16[]})
        n120 = local write "枚举"(enum16{"读取", "写入", "读取参数"}."写入" ("枚举")) -> ()
        n121 = Enqueue Element(queue=w230, element=w233) -> ()  [unwired: 2 in, 3 out]
      }
      event "空白测试": Value Change {
        n122 = event-data() -> ()  [unwired: 1 in, 6 out]
        n123 = local write "启动测量模式"(T1."空白测试" ("启动测量模式")) -> ()
        n124 = Bundle By Name(cluster=cluster{"starting address":u16, "values":u16[]} {"starting address"=0, "values"=[]} ("元素"), "starting address"=u16 4608, "values"=u16[] [5]) -> (w240:cluster{"starting address":u16, "values":u16[]})
        n125 = local write "枚举"(enum16{"读取", "写入", "读取参数"}."写入" ("枚举")) -> ()
        n126 = Enqueue Element(queue=w237, element=w240) -> ()  [unwired: 2 in, 3 out]
      }
      event "空白校准": Value Change {
        n127 = event-data() -> ()  [unwired: 1 in, 6 out]
        n128 = local write "启动测量模式"(T1."空白校准" ("启动测量模式")) -> ()
        n129 = Bundle By Name(cluster=cluster{"starting address":u16, "values":u16[]} {"starting address"=0, "values"=[]} ("元素"), "starting address"=u16 4608, "values"=u16[] [8]) -> (w247:cluster{"starting address":u16, "values":u16[]})
        n130 = local write "枚举"(enum16{"读取", "写入", "读取参数"}."写入" ("枚举")) -> ()
        n131 = Enqueue Element(queue=w244, element=w247) -> ()  [unwired: 2 in, 3 out]
      }
      event "标样校准": Value Change {
        n132 = event-data() -> ()  [unwired: 1 in, 6 out]
        n133 = local write "启动测量模式"(T1."标样校准" ("启动测量模式")) -> ()
        n134 = Bundle By Name(cluster=cluster{"starting address":u16, "values":u16[]} {"starting address"=0, "values"=[]} ("元素"), "starting address"=u16 4608, "values"=u16[] [9]) -> (w254:cluster{"starting address":u16, "values":u16[]})
        n135 = local write "枚举"(enum16{"读取", "写入", "读取参数"}."写入" ("枚举")) -> ()
        n136 = Enqueue Element(queue=w251, element=w254) -> ()  [unwired: 2 in, 3 out]
      }
      event "停止": Value Change {
        n137 = event-data() -> ()  [unwired: 1 in, 6 out]
        n138 = Cancel Notification(0:w259) -> (8:w258:refnum<notifier>)  [unwired: 1 in, 2 out]
        n139 = local write "启动测量模式"(T1."空闲" ("启动测量模式")) -> ()
        n140 = Send Notification(notification=TRUE ("通知"), notifier=w258) -> ()  [unwired: 1 in, 2 out]
        n141 = Bundle By Name(cluster=cluster{"starting address":u16, "values":u16[]} {"starting address"=0, "values"=[]} ("元素"), "starting address"=u16 4608, "values"=u16[] [12]) -> (w264:cluster{"starting address":u16, "values":u16[]})
        n142 = local write "枚举"(enum16{"读取", "写入", "读取参数"}."写入" ("枚举")) -> ()
        n143 = Enqueue Element(queue=w261, element=w264) -> ()  [unwired: 2 in, 3 out]
      }
      event "保存KB值": Value Change {
        n144 = event-data() -> ()  [unwired: 1 in, 6 out]
        n145 = local read "曲线斜率B"() -> (w267:sgl)
        n146 = local read "曲线斜率K"() -> (w268:sgl)
        n147 = Build Array(w268, w267) -> (w266:sgl[])
        n148 = call "FloatToHex.vi"("浮点数"=w266) -> ("DCBA整形输出"=w269:u16[])  [unwired: 10 in]
        n149 = Bundle By Name(cluster=cluster{"starting address":u16, "values":u16[]} {"starting address"=0, "values"=[]} ("元素"), "starting address"=u16 4263, "values"=w269) -> (w271:cluster{"starting address":u16, "values":u16[]})
        n150 = Enqueue Element(queue=w273, element=w271) -> ()  [unwired: 2 in, 3 out]
        n151 = local write "枚举"(enum16{"读取", "写入", "读取参数"}."写入" ("枚举")) -> ()
      }
      event "写入消解温度时长": Value Change {
        n152 = event-data() -> ()  [unwired: 1 in, 6 out]
        n153 = local read "消解时长"() -> (w276:u16)
        n154 = local read "消解温度"() -> (w277:u16)
        n155 = Build Array(w277, w276) -> (w275:u16[])
        n156 = call "WordToHex.vi"("WORD"=w275) -> ("数组"=w278:u16[])  [unwired: 10 in]
        n157 = Bundle By Name(cluster=cluster{"starting address":u16, "values":u16[]} {"starting address"=0, "values"=[]} ("元素"), "starting address"=u16 4257, "values"=w278) -> (w281:cluster{"starting address":u16, "values":u16[]})
        n158 = Enqueue Element(queue=w279, element=w281) -> ()  [unwired: 2 in, 3 out]
      }
      event "校时": Value Change {
        n159 = event-data() -> ()  [unwired: 1 in, 6 out]
        n160 = Get Date/Time In Seconds() -> (seconds since 1Jan1904=w289:timestamp)
        n161 = Build Array(w289) -> (w288:timestamp[])
        n162 = call "DateToHex.vi"("DATE"=w288) -> ("数组"=w286:u16[])  [unwired: 10 in]
        n163 = Insert Into Array(array=u16[] [13] ("values"), index=1 ("索引"), new element=w286) -> (w284:u16[])
        n164 = local write "枚举"(enum16{"读取", "写入", "读取参数"}."写入" ("枚举")) -> ()
        n165 = Bundle By Name(cluster=cluster{"starting address":u16, "values":u16[]} {"starting address"=0, "values"=[]} ("元素"), "starting address"=u16 4608, "values"=w284) -> (w292:cluster{"starting address":u16, "values":u16[]})
        n166 = Enqueue Element(queue=w290, element=w292) -> ()  [unwired: 2 in, 3 out]
      }
      event "设置": Value Change {
        n167 = event-data() -> ()  [unwired: 1 in, 6 out]
        n168 = property on="窗格" class="Pane"("Origin"=T7 {"Horizontal"=0, "Vertical"=728} ("原点")) -> ()  [unwired: 2 in, 2 out]
        n169 = flat-sequence {
          tunnel: w294 -> [w296]
          frame #0 {
            n170 = Bundle By Name(cluster=T6 {"starting address"=0, "number of holding registers"=0} ("元素"), "starting address"=u16 4256, "number of holding registers"=u16 19) -> (w300:T6)
            n171 = Enqueue Element(queue=w296, element=w300) -> ()  [unwired: 2 in, 3 out]
          }
          frame #1 {
            n172 = local write "枚举"(enum16{"读取", "写入", "读取参数"}."读取参数" ("枚举")) -> ()
          }
        }
      }
      event "返回": Value Change {
        n173 = event-data() -> ()  [unwired: 1 in, 6 out]
        n174 = property on="窗格" class="Pane"("Origin"=T7 {"Horizontal"=0, "Vertical"=0} ("原点")) -> ()  [unwired: 2 in, 2 out]
        n175 = property on="写入消解温度时长" class="Bool"("Visible"=FALSE ("可见")) -> ()  [unwired: 2 in, 2 out]
      }
      event "曲线斜率K", "曲线斜率B", "消解温度", "消解时长": Mouse Down {
        n176 = event-data() -> ("CtlRef"=w306:refnum<vi>)  [unwired: 1 in, 7 out]
        n177 = property class="DigNum"(reference=w306) -> (reference out=w307:refnum<vi>, "Value"=w305:variant)  [unwired: 1 in, 1 out]
        n178 = Variant To Data(Variant=w305) -> (data=w304:sgl)  [unwired: 2 in, 1 out]
        n179 = call "CODCR数字键盘.vi"("OldNumber"=w304) -> ("NewNumber"=w308:sgl)
        n180 = property class="DigNum"(reference=w307, "Value"=w308) -> ()  [unwired: 1 in, 2 out]
      }
      event "隐藏按钮": Value Change {
        n181 = event-data() -> ()  [unwired: 1 in, 6 out]
        n182 = property on="写入消解温度时长" class="Bool"("Visible"=TRUE ("可见")) -> ()  [unwired: 2 in, 2 out]
      }
    }
  }
  "COM口" <- "VISA Resource"
